vi "metal particle analysis.vi"() -> ()   [LabVIEW 2013]
panel:
  out "Particle Measurements(pixels)":dbl[][](array[numeric]) format="%.2f"
  out "Number of Particles":i32
  in  "Number of Images":i32=4
  out "Image Out":T1(plugin-control)
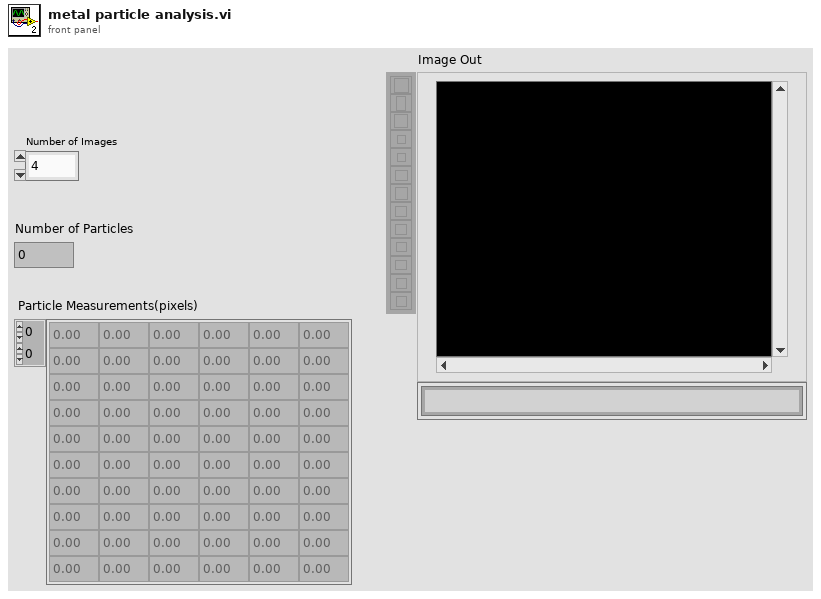
[diagram p1: front panel]
types:
  T1 = typedef "IMAQ Image.ctl" = refnum<image>
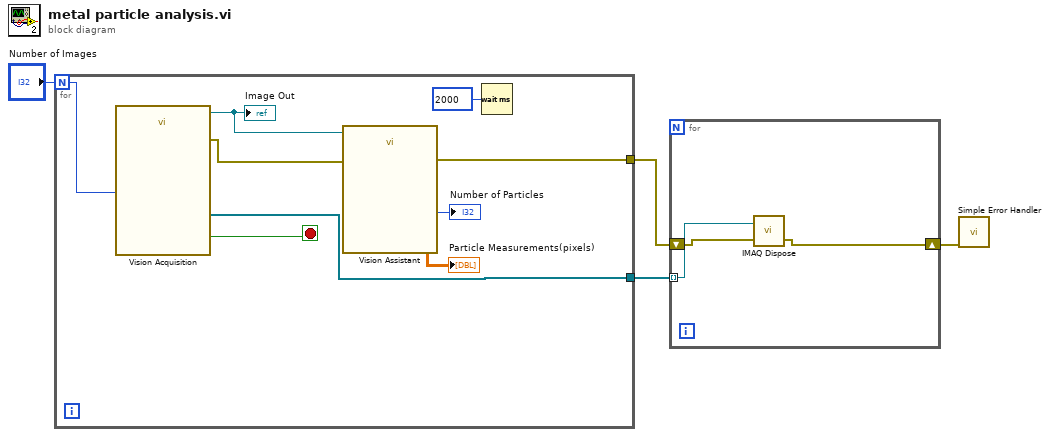
[diagram p0: block diagram]
diagram:
  n1 = for {
    N: "Number of Images" -> [w13]
    tunnel: [w6] -> w3
    tunnel: [w5] -> w2
    stop <- w12 stop-if-true
    n2 = call "Vision Acquisition"("Number of Images"=w13) -> ("Image Out"=w11:T1, "All Images Out"=w6:T1[], "Stopped"=w12:bool, "error out"=w10:errorcluster)  [unwired: 23 in]
    "Image Out" <- w11
    n3 = call "Vision Assistant"("Image In"=w11, "error in"=w10) -> ("Number of Particles (Particle Analysis 1)"=→"Number of Particles":i32, "Particle Measurements (Pixels) (Particle Analysis 1)"=→"Particle Measurements(pixels)":dbl[][], "error out"=w5:errorcluster)  [unwired: 22 in, 1 out]
    n4 = Wait (ms)(milliseconds to wait=u32 2000 ("等待时间（毫秒）")) -> ()  [unwired: 1 out]
  }
  n5 = for {
    tunnel: w3 -> [w15] mode=indexing
    shift-right: [w14] -> w1
    shift-left: w2 -> [w16]
    n6 = call "IMAQ Dispose"("Image"=w15, "error in (no error)"=w16) -> ("error out"=w14:errorcluster)  [unwired: 4 in]
  }
  n7 = call <vilib>:"Simple Error Handler.vi"("error in (no error)"=w1) -> ()  [unwired: 4 in, 5 out]
